vi "Find Rootmost Partial Matches.vi"(8 "error in":errorcluster, 10 "Branch Name Pattern":string, 11 "Tree in":refnum<class "Tree.lvclass">) -> (0 "error out":errorcluster, 1 "Found?":bool, 2 "Root Most Partial Matches":refnum<class "Tree.lvclass">[](array[class]), 3 "Tree out":refnum<class "Tree.lvclass">)   [LabVIEW 2019, in "Tree.lvclass"]
uses:
  Tree.lvclass
  Tree.lvclass/Tree.ctl
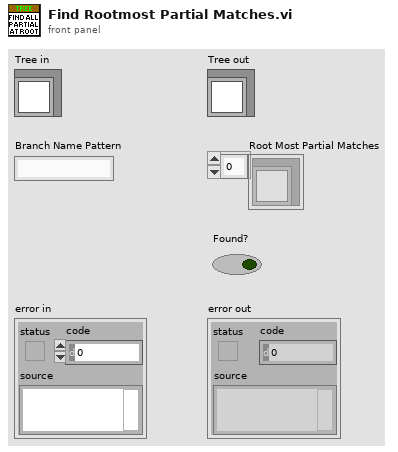
[diagram p1: front panel]
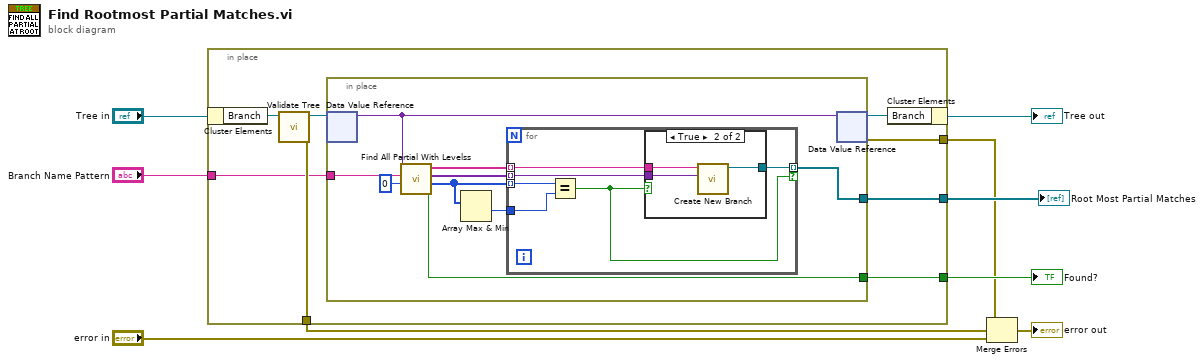
[diagram p0: block diagram]
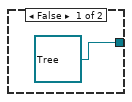
[diagram p2: hidden frame]
diagram:
  n1 = in-place {
    in-place-border: [w16] -> w1
    in-place-border: [w13] -> w5
    in-place-border: "Branch Name Pattern" -> [w12]
    in-place-border: [w11] -> w3
    in-place-border: [w10] -> w2
    n2 = in-place-cluster #1("Tree in") -> ("Branch"=w15:refnum<data-value>)
    n3 = call "Validate Tree.vi"("Branch Reference In"=w15) -> ("error out"=w13:errorcluster, "Branch Reference Out"=w14:refnum<data-value>)  [unwired: 9 in]
    n4 = in-place {
      in-place-border: w12 -> [w25]
      in-place-border: [w19] -> w11
      in-place-border: [w18] -> w10
      n5 = in-place-dvr #2(w14) -> (w26:variant)  [unwired: 1 out]
      n6 = call "Find All Partial With Levelss.vi"("Level"=0, "Name"=w25, "Tree"=w26) -> ("Found?"=w18:bool, "Levels"=w20:i32[], "Match"=w22:variant[], "Node Name"=w23:string[])  [unwired: 5 in]
      n7 = Array Max & Min(array=w20) -> (min value=w21:i32)  [unwired: 3 out]
      n8 = for {
        tunnel: w23 -> [w29] mode=indexing
        tunnel: w22 -> [w30] mode=indexing
        tunnel: w21 -> [w31]
        tunnel: w20 -> [w32] mode=indexing
        tunnel: [w28] -> w19 mode=indexing if=w27
        n9 = Equal?(x=w32, y=w31) -> (x = y?=w27:bool)
        n10 = case shown="True" w27 {
          tunnel: w30 -> [_ w36]
          tunnel: [refnum<class "Tree.lvclass"> refnum ("Tree out") w35] -> w28
          tunnel: w29 -> [_ w34]
          frame False {
          }
          frame True {
            n11 = call "Create New Branch.vi"("Branch Data"=w36, "Name"=w34) -> ("Tree out"=w35:refnum<class "Tree.lvclass">)  [unwired: 8 in, 1 out]
          }
        }
      }
      n12 = in-place-dvr #2(w26) -> (w17:refnum<data-value>, w16:errorcluster)
    }
    n13 = in-place-cluster #1("Branch"=w17) -> (→"Tree out":refnum<class "Tree.lvclass">)
  }
  "Found?" <- w2
  "Root Most Partial Matches" <- w3
  n14 = Merge Errors(w1, w5, "error in") -> (→"error out":errorcluster)
